vi "Pneumatics Control Simulator.vi"() -> ()   [LabVIEW 2015]
uses:
  <userlib>/836 Library/Pneumatics/Pneumatics/Pneumatic Configuration.ctl
  <userlib>/836 Library/Pneumatics/Common/Feedback Typedef.ctl
  <vilib>/Rock Robotics/WPI/Solenoid/WPI_SolenoidChannel.ctl
  <vilib>/Rock Robotics/WPI/Solenoid/WPI_SolenoidOpenSingle.vi
  <userlib>/836 Library/Pneumatics/Pneumatics/2-Position Solenoid Control.vi
panel:
  in  "Initial Position":bool=TRUE
  in  "Feedback":T1
  in  "Pneumatic Configuration":T2={"Time Forward (ms)"=6, "Time Back (ms)"=1, "Digital Forward Time (ms)"=3000, "Digital Backward Time (ms)"=5000, "Analog Forward Settling Time (ms)"=4000, "Analog Backward Settling Time (ms)"=2000, "Analog Forward Threshold"=4.0, "Analog Backward Threshold"=1.0}
  in  "Action":T3(ring)=enum."Toggle"
  out "Action Complete":bool
  out "Forward":bool
  in  "Sensor Analog Status":sgl(knob)=5.0 scale=0.0..5.0
  in  "Sensor Digital Status":bool
  in  "Step":bool
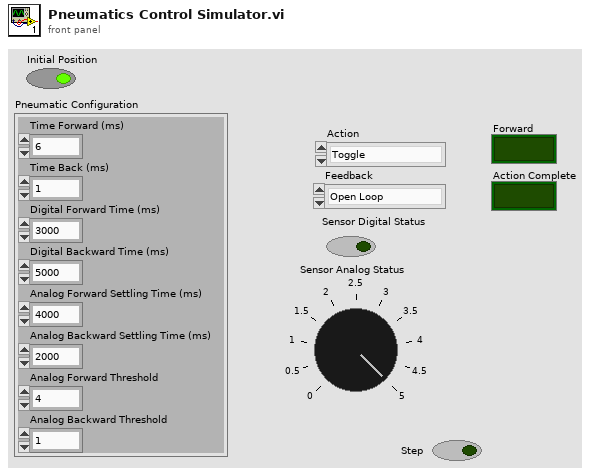
[diagram p1: front panel]
types:
  T1 = typedef "Feedback Typedef.ctl" = enum16{"Open Loop", "Analog", "Digital", "Timed", "Digital Timeout"}
  T2 = typedef "Pneumatic Configuration.ctl" = cluster{"Time Forward (ms)":u32, "Time Back (ms)":u32, "Digital Forward Time (ms)":u32, "Digital Backward Time (ms)":u32, "Analog Forward Settling Time (ms)":u32, "Analog Backward Settling Time (ms)":u32, "Analog Forward Threshold":sgl, "Analog Backward Threshold":sgl}
  T3 = enum16{"Forward", "Back", "Toggle", "Status", "Off"}
  T4 = typedef "WPI_SolenoidChannel.ctl" = enum8{"Solenoid 0", "Solenoid 1", "Solenoid 2", "Solenoid 3", "Solenoid 4", "Solenoid 5", "Solenoid 6", "Solenoid 7", "Invalid"}
  T5 = typedef "WPI_SolenoidDevRef.ctl" = cluster{"DevStatus":errorcluster, "Pneumatics Control Module":u8, "Forward Solenoid Channel":T4, "Reverse Solenoid Channel":T4}
  T6 = typedef "836_PneumaticsDevRef.ctl" = cluster{"Pneumatic State Reference":refnum<data-value>, "SolenoidDevRef":T5, "Pneumatic Configuration reference":refnum<data-value>}
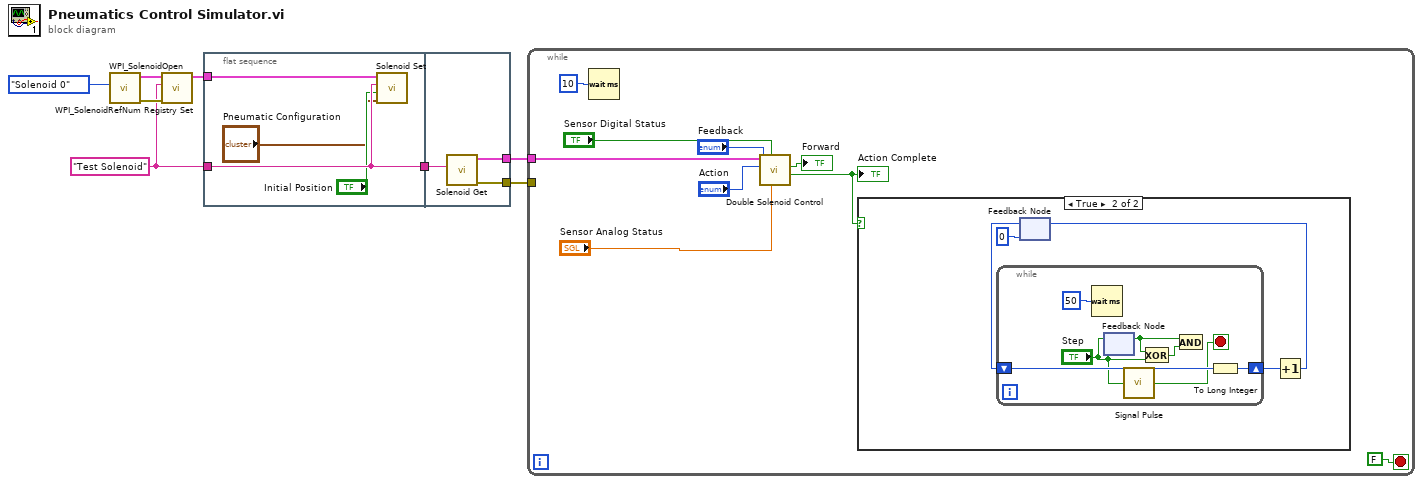
[diagram p0: block diagram]
diagram:
  w2 = "Test Solenoid" ("DevRef")
  n1 = call-poly <vilib>:"WPI_SolenoidOpen.vi"("Solenoid Channel"=WPI_SolenoidChannel."Solenoid 0") -> ("error out"=w4:errorcluster, "SolenoidDevRef"=w5:T5)  [unwired: 9 in]
  n2 = call <vilib>:"WPI_SolenoidRefNum Registry Set.vi"("error in (no error)"=w4, "refnum name"=w2, "SolenoidDevRef"=w5) -> ("SolenoidDevRef"=w3:T5)  [unwired: 7 in, 1 out]
  n3 = flat-sequence {
    tunnel: w2 -> [w12]
    tunnel: [w12] -> w6
    tunnel: w3 -> [w10]
    tunnel: [w15] -> w8
    tunnel: [w14] -> w7
    tunnel: w6 -> [w13]
    frame #0 {
      n4 = call <userlib>:"Solenoid Set.vi"("Pneumatic Configuration"="Pneumatic Configuration", "Initial Position"="Initial Position", "DevRef"=w12, "SolenoidDevRef"=w10) -> ()  [unwired: 7 in, 1 out]
    }
    frame #1 {
      n5 = call <userlib>:"Solenoid Get.vi"("DevRef"=w13) -> ("Error Out"=w14:errorcluster, "PneumaticsDevRefOut"=w15:T6)  [unwired: 9 in]
    }
  }
  n6 = while {
    tunnel: w8 -> [w17]
    tunnel: w7 -> [_]
    stop <- FALSE stop-if-true
    n7 = Wait (ms)(milliseconds to wait=u32 10) -> ()  [unwired: 1 out]
    n8 = call-poly <userlib>:"Double Solenoid Control.vi"("Sensor Analog Status"="Sensor Analog Status", "Sensor Digital Status"="Sensor Digital Status", "Feedback"="Feedback", "Action"="Action", "PneumaticsDevRefIn"=w17) -> ("Action Complete"=w18:bool, "Forward"=→"Forward":bool)  [unwired: 4 in, 1 out]
    "Action Complete" <- w18
    n9 = case shown="True" w18 {
      frame False {
      }
      frame True {
        n10 = feedback #1(0) -> (w26:i32)
        n11 = while {
          shift-right: [w33] -> w28
          shift-left: w26 -> [w32]
          stop <- w29 stop-if-true
          n12 = Wait (ms)(milliseconds to wait=u32 50) -> ()  [unwired: 1 out]
          n13 = feedback-in #2("Step") -> ()
          n14 = feedback #2() -> (w34:bool)  [unwired: 1 in]
          n15 = call <userlib>:"Signal Pulse.vi"("Input"="Step") -> ("Output"=w29:bool)
          n16 = Exclusive Or(1:"Step", 2:w34) -> (0:w35:bool)
          n17 = And(x=w34, y=w35) -> ()  [unwired: 1 out]
          n18 = To Long Integer(number=w32) -> (32bit integer=w33:i32)
        }
        n19 = Increment(x=w28) -> (x+1=w27:i32)
        n20 = feedback-in #1(w27) -> ()
      }
    }
  }
